vi "Build Error Message.vi"(8 "error in (no error)":errorcluster, 10 "Data":variant, 11 "Arg":string) -> (0 "error out":errorcluster)   [LabVIEW 2020, in "VI Properties Editor.lvlib"]
doc: "Appends text to the end of the error message indicating the State/Arg where the error occurred, and works in conjunction with <B>Producer Loop Guard Clause.vi</B> to catch and handle any errors that may have occurred in the Producer Loop."
uses:
  VI Properties Editor.lvlib
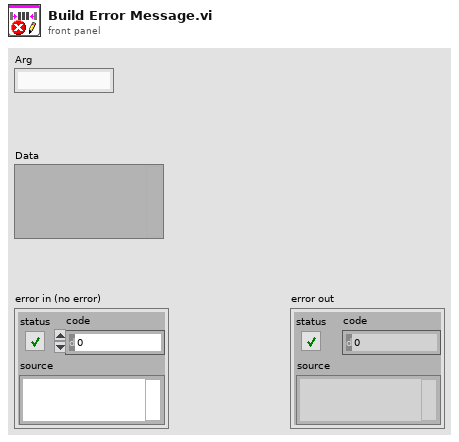
[diagram p1: front panel]
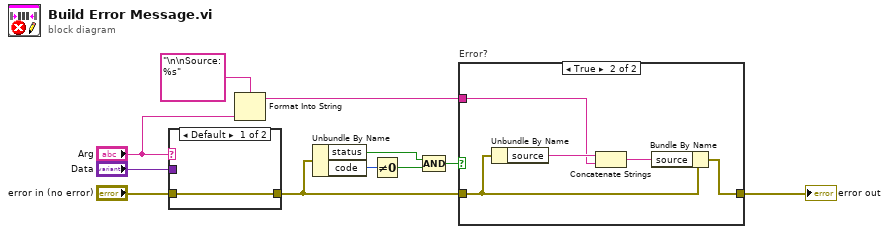
[diagram p0: block diagram]
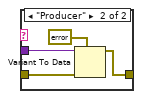
[diagram p2: hidden frame]
diagram:
  n1 = case shown="Default" "Arg" {
    tunnel: "Data" -> [_ w15]
    tunnel: "error in (no error)" -> [w12 w16]
    tunnel: [w12 w13] -> w3
    frame Default {
    }
    frame "Producer" {
      n2 = Variant To Data(error in=w16, type=errorcluster {"status"=FALSE, "code"=0, "source"=""} ("error out"), Variant=w15) -> (data=w13:errorcluster)  [unwired: 1 out]
    }
  }
  n3 = Format Into String(format string="\n\nSource: %s", "Arg") -> (resulting string=w2:string)  [unwired: 2 in, 1 out]
  n4 = Unbundle By Name(w3) -> ("status"=w4:bool, "code"=w7:i32)
  n5 = Not Equal To 0?(x=w7) -> (x != 0?=w6:bool)
  n6 = Compound Arithmetic op=AND(w4, w6) -> (w5:bool)
  n7 = case "Error?" shown="True" w5 {
    tunnel: w3 -> [w17 w22]
    tunnel: [w17 w21] -> w1
    tunnel: w2 -> [_ w18]
    frame False {
    }
    frame True {
      n8 = Unbundle By Name(w22) -> ("source"=w20:string)
      n9 = Concatenate Strings(w20, w18) -> (w19:string)
      n10 = Bundle By Name(cluster=w22, "source"=w19) -> (w21:errorcluster)
    }
  }
  "error out" <- w1
